vi "Explain.vi"(8 "error in (no error)":errorcluster, 10 "Verbose Explanation":string, 11 "Test Assert in":refnum<class "Test Assert.lvclass">) -> (0 "error out":errorcluster, 3 "Test Assert out":refnum<class "Test Assert.lvclass">)   [LabVIEW 2013, in "Caraya.lvlib" / "Test Assert.lvclass"]
uses:
  Test Assert.lvclass
  Assert/Assert.lvclass
  Test Assert.lvclass/Test Assert.ctl
  Test Manager/Test Manager.lvclass
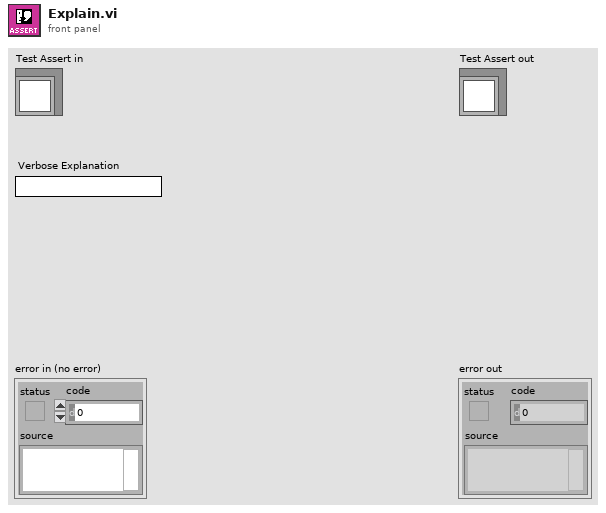
[diagram p1: front panel]
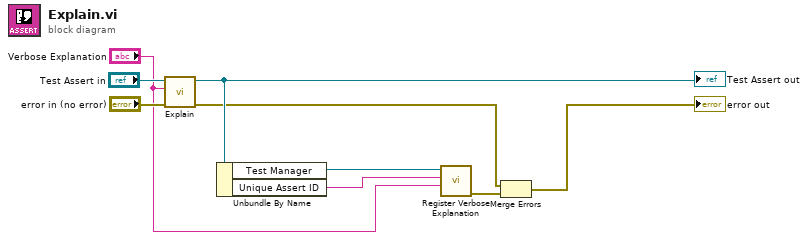
[diagram p0: block diagram]
diagram:
  n1 = call-parent "Explain.vi"("error in (no error)"="error in (no error)", "Verbose Explanation"="Verbose Explanation", "Assert in"="Test Assert in") -> ("error out"=w2:errorcluster, "Assert out"=w7:refnum<class "Test Assert.lvclass">)  [unwired: 7 in]
  "Test Assert out" <- w7
  n2 = Unbundle By Name(w7) -> ("Test Manager"=w6:refnum<class "Test Manager.lvclass">, "Unique Assert ID"=w5:string)
  n3 = call-dynamic "Register Verbose Explanation.vi"("Explanation"="Verbose Explanation", "Unique ID"=w5, "Test Manager in"=w6) -> ("error out"=w3:errorcluster)  [unwired: 7 in, 1 out]
  n4 = Merge Errors(w2, w3) -> (→"error out":errorcluster)
